vi "Choose_nest.vi"() -> ()   [LabVIEW 2023]
panel:
  in  "Nest":u16(ring) items=["Nest 0", "Nest 1", "Nest 2", "Nest 3", "Nest 4", "Nest 5"]
  out "error out":errorcluster
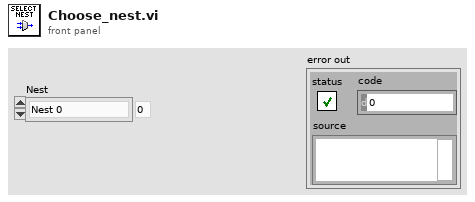
[diagram p1: front panel]
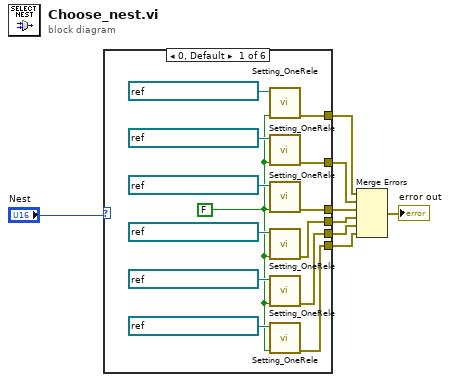
[diagram p0: block diagram]
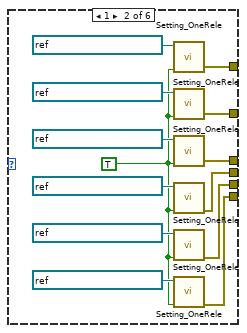
[diagram p2: hidden frame]
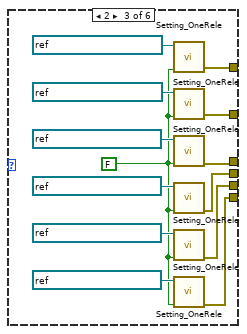
[diagram p3: hidden frame]
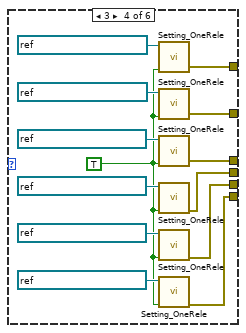
[diagram p4: hidden frame]
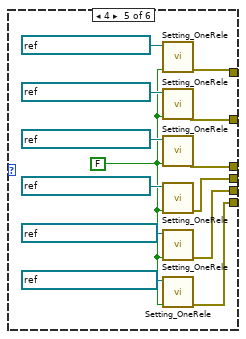
[diagram p5: hidden frame]
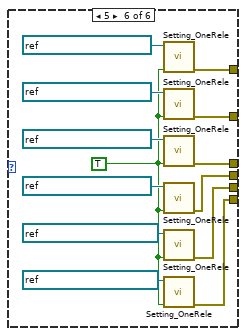
[diagram p6: hidden frame]
diagram:
  n1 = case shown="0, Default" "Nest" {
    tunnel: [w15 w27 w40 w53 w66 w74] -> w8
    tunnel: [w14 w26 w39 w52 w65 w75] -> w7
    tunnel: [w13 w25 w35 w51 w64 w76] -> w6
    tunnel: [w12 w24 w36 w48 w61 w77] -> w5
    tunnel: [w11 w23 w37 w49 w62 w78] -> w4
    tunnel: [w10 w22 w38 w50 w63 w79] -> w3
    frame 0, Default {
      w9 = FALSE
      n2 = call "Setting_OneRele.vi"("data"=w9, "line"=refnum<k21> "Dev0/1stPortA/Do0") -> ("error out"=w15:errorcluster)  [unwired: 9 in]
      n3 = call "Setting_OneRele.vi"("data"=w9, "line"=refnum<k21> "Dev0/1stPortA/Do1") -> ("error out"=w14:errorcluster)  [unwired: 9 in]
      n4 = call "Setting_OneRele.vi"("data"=w9, "line"=refnum<k21> "Dev0/1stPortA/Do2") -> ("error out"=w13:errorcluster)  [unwired: 9 in]
      n5 = call "Setting_OneRele.vi"("data"=w9, "line"=refnum<k21> "Dev0/1stPortA/Do3") -> ("error out"=w12:errorcluster)  [unwired: 9 in]
      n6 = call "Setting_OneRele.vi"("data"=w9, "line"=refnum<k21> "Dev0/1stPortA/Do4") -> ("error out"=w11:errorcluster)  [unwired: 9 in]
      n7 = call "Setting_OneRele.vi"("data"=w9, "line"=refnum<k21> "Dev0/1stPortA/Do5") -> ("error out"=w10:errorcluster)  [unwired: 9 in]
    }
    frame 1 {
      w28 = TRUE
      n8 = call "Setting_OneRele.vi"("data"=w28, "line"=refnum<k21> "Dev0/1stPortA/Do0") -> ("error out"=w27:errorcluster)  [unwired: 9 in]
      n9 = call "Setting_OneRele.vi"("data"=w28, "line"=refnum<k21> "Dev0/1stPortA/Do1") -> ("error out"=w26:errorcluster)  [unwired: 9 in]
      n10 = call "Setting_OneRele.vi"("data"=w28, "line"=refnum<k21> "Dev0/1stPortA/Do2") -> ("error out"=w25:errorcluster)  [unwired: 9 in]
      n11 = call "Setting_OneRele.vi"("data"=w28, "line"=refnum<k21> "Dev0/1stPortA/Do3") -> ("error out"=w24:errorcluster)  [unwired: 9 in]
      n12 = call "Setting_OneRele.vi"("data"=w28, "line"=refnum<k21> "Dev0/1stPortA/Do4") -> ("error out"=w23:errorcluster)  [unwired: 9 in]
      n13 = call "Setting_OneRele.vi"("data"=w28, "line"=refnum<k21> "Dev0/1stPortA/Do5") -> ("error out"=w22:errorcluster)  [unwired: 9 in]
    }
    frame 2 {
      w41 = FALSE
      n14 = call "Setting_OneRele.vi"("data"=w41, "line"=refnum<k21> "Dev0/1stPortA/Do6") -> ("error out"=w40:errorcluster)  [unwired: 9 in]
      n15 = call "Setting_OneRele.vi"("data"=w41, "line"=refnum<k21> "Dev0/1stPortA/Do7") -> ("error out"=w39:errorcluster)  [unwired: 9 in]
      n16 = call "Setting_OneRele.vi"("data"=w41, "line"=refnum<k21> "Dev0/1stPortB/Do0") -> ("error out"=w35:errorcluster)  [unwired: 9 in]
      n17 = call "Setting_OneRele.vi"("data"=w41, "line"=refnum<k21> "Dev0/1stPortB/Do1") -> ("error out"=w36:errorcluster)  [unwired: 9 in]
      n18 = call "Setting_OneRele.vi"("data"=w41, "line"=refnum<k21> "Dev0/1stPortB/Do2") -> ("error out"=w37:errorcluster)  [unwired: 9 in]
      n19 = call "Setting_OneRele.vi"("data"=w41, "line"=refnum<k21> "Dev0/1stPortB/Do3") -> ("error out"=w38:errorcluster)  [unwired: 9 in]
    }
    frame 3 {
      w54 = TRUE
      n20 = call "Setting_OneRele.vi"("data"=w54, "line"=refnum<k21> "Dev0/1stPortA/Do6") -> ("error out"=w53:errorcluster)  [unwired: 9 in]
      n21 = call "Setting_OneRele.vi"("data"=w54, "line"=refnum<k21> "Dev0/1stPortA/Do7") -> ("error out"=w52:errorcluster)  [unwired: 9 in]
      n22 = call "Setting_OneRele.vi"("data"=w54, "line"=refnum<k21> "Dev0/1stPortB/Do0") -> ("error out"=w51:errorcluster)  [unwired: 9 in]
      n23 = call "Setting_OneRele.vi"("data"=w54, "line"=refnum<k21> "Dev0/1stPortB/Do1") -> ("error out"=w48:errorcluster)  [unwired: 9 in]
      n24 = call "Setting_OneRele.vi"("data"=w54, "line"=refnum<k21> "Dev0/1stPortB/Do2") -> ("error out"=w49:errorcluster)  [unwired: 9 in]
      n25 = call "Setting_OneRele.vi"("data"=w54, "line"=refnum<k21> "Dev0/1stPortB/Do3") -> ("error out"=w50:errorcluster)  [unwired: 9 in]
    }
    frame 4 {
      w67 = FALSE
      n26 = call "Setting_OneRele.vi"("data"=w67, "line"=refnum<k21> "Dev0/1stPortB/Do4") -> ("error out"=w66:errorcluster)  [unwired: 9 in]
      n27 = call "Setting_OneRele.vi"("data"=w67, "line"=refnum<k21> "Dev0/1stPortB/Do5") -> ("error out"=w65:errorcluster)  [unwired: 9 in]
      n28 = call "Setting_OneRele.vi"("data"=w67, "line"=refnum<k21> "Dev0/1stPortB/Do6") -> ("error out"=w64:errorcluster)  [unwired: 9 in]
      n29 = call "Setting_OneRele.vi"("data"=w67, "line"=refnum<k21> "Dev0/1stPortB/Do7") -> ("error out"=w61:errorcluster)  [unwired: 9 in]
      n30 = call "Setting_OneRele.vi"("data"=w67, "line"=refnum<k21> "Dev0/1stPortCL/Do0") -> ("error out"=w62:errorcluster)  [unwired: 9 in]
      n31 = call "Setting_OneRele.vi"("data"=w67, "line"=refnum<k21> "Dev0/1stPortCL/Do1") -> ("error out"=w63:errorcluster)  [unwired: 9 in]
    }
    frame 5 {
      w80 = TRUE
      n32 = call "Setting_OneRele.vi"("data"=w80, "line"=refnum<k21> "Dev0/1stPortB/Do4") -> ("error out"=w74:errorcluster)  [unwired: 9 in]
      n33 = call "Setting_OneRele.vi"("data"=w80, "line"=refnum<k21> "Dev0/1stPortB/Do5") -> ("error out"=w75:errorcluster)  [unwired: 9 in]
      n34 = call "Setting_OneRele.vi"("data"=w80, "line"=refnum<k21> "Dev0/1stPortB/Do6") -> ("error out"=w76:errorcluster)  [unwired: 9 in]
      n35 = call "Setting_OneRele.vi"("data"=w80, "line"=refnum<k21> "Dev0/1stPortB/Do7") -> ("error out"=w77:errorcluster)  [unwired: 9 in]
      n36 = call "Setting_OneRele.vi"("data"=w80, "line"=refnum<k21> "Dev0/1stPortCL/Do0") -> ("error out"=w78:errorcluster)  [unwired: 9 in]
      n37 = call "Setting_OneRele.vi"("data"=w80, "line"=refnum<k21> "Dev0/1stPortCL/Do1") -> ("error out"=w79:errorcluster)  [unwired: 9 in]
    }
  }
  n38 = Merge Errors(w8, w7, w6, w5, w4, w3) -> (→"error out":errorcluster)
